vi "myRIO_BRig_FPGA_v3,41__PortC__v2.vi"() -> ()   [LabVIEW 2014]
uses:
  <vilib>/rvi/FXPMathLib/FxpDiv/subVIs/nifxpmath_Div_SimConfig.ctl
  <vilib>/rvi/FXPMathLib/FxpSinAndCos/subVIs/nifxpmath_SinAndCos_SimConfig.ctl
  <vilib>/rvi/FXPMathLib/FxpDiv/simVIs/DllFxpDivTemp_sub.vi
  <vilib>/rvi/FXPMathLib/FxpSinAndCos/simVIs/DllFxpSinAndCosTemp_sub.vi
  <vilib>/rvi/Emulation/niFpgaGetClockAttributes.vi
  <vilib>/rvi/Emulation/niFpgaSctlEmulationGetInTimedLoop.vi
  <vilib>/rvi/Emulation/niFpgaEmulationReportErrorSimple.vi
  <vilib>/rvi/eio/common/nirviEmuTemplateMethod_errors.vi
  <vilib>/rvi/Emulation/niFpgaCriticalErrorInLSC.vi
  <vilib>/rvi/FXPMathLib/FxpDiv/XNode/nifxpmath_Div.xnode
  <vilib>/rvi/FXPMathLib/FxpMul/XNode/nifxpmath_Multiplier.xnode
  <vilib>/rvi/FXPMathLib/FxpSinAndCos/XNode/nifxpmath_SinAndCos.xnode
  <vilib>/rvi/FXPMathLib/FxpSub/XNode/nifxpmath_Sub.xnode
  <vilib>/eio/EIONode/EIONode.xnode
  <vilib>/rvi/FXPMathLib/sim/FxpSim.dll
panel:
  in  "laser_Nshutter":u32=100
  in  "AnaOut_0":i16
  in  "laser_Nvalley":u32=100
  in  "laser_Npeak":u32=100
  in  "laserledMTrig":bool
  in  "laser_selWro_Ntotal":u32=100
  in  "laser_selWro_NDelay":u32
  in  "laser_selRew_Ntotal":u32=100
  in  "laser_selRew_Ndelay":u32
  in  "laserResponse_reward_LED":bool
  in  "laserResponse_wrong_LED":bool
  out "SelectWrong":bool
  out "SelectReward":bool
  in  "laserResponse_wrong":bool
  in  "laserResponse_reward":bool
  in  "Left(F)_or_Right(T)":bool
  in  "ignoreWrong":bool
  in  "SelectionState":bool
  in  "laserMTrig":bool
  in  "FPGA_Stop":bool
  in  "audioTrigger_L":bool
  in  "audioTrigger_R":bool
  in  "audioFreq_L_Hz":u16=1000 min=1000 max=14000 step=1000
  in  "audioAmp_L":u16=1 min=1 max=32767 step=1
  in  "audioFreq_R_Hz":u16=1000 min=1000 max=14000 step=1000
  in  "audioAmp_R":u16=1 min=1 max=32767 step=1
  in  "A3_SL":bool
  in  "A1_SR":bool
  in  "Counts_Reset":bool
  out "A4_LickR":u32
  out "A2_LickL":u32
  in  "A6_Act":bool
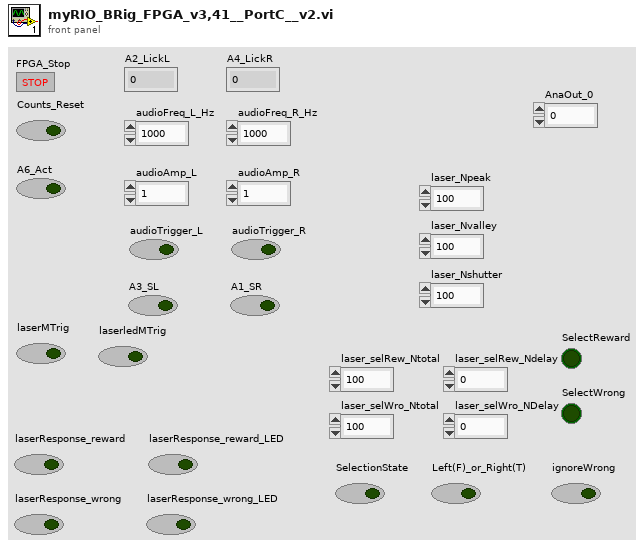
[diagram p1: front panel]
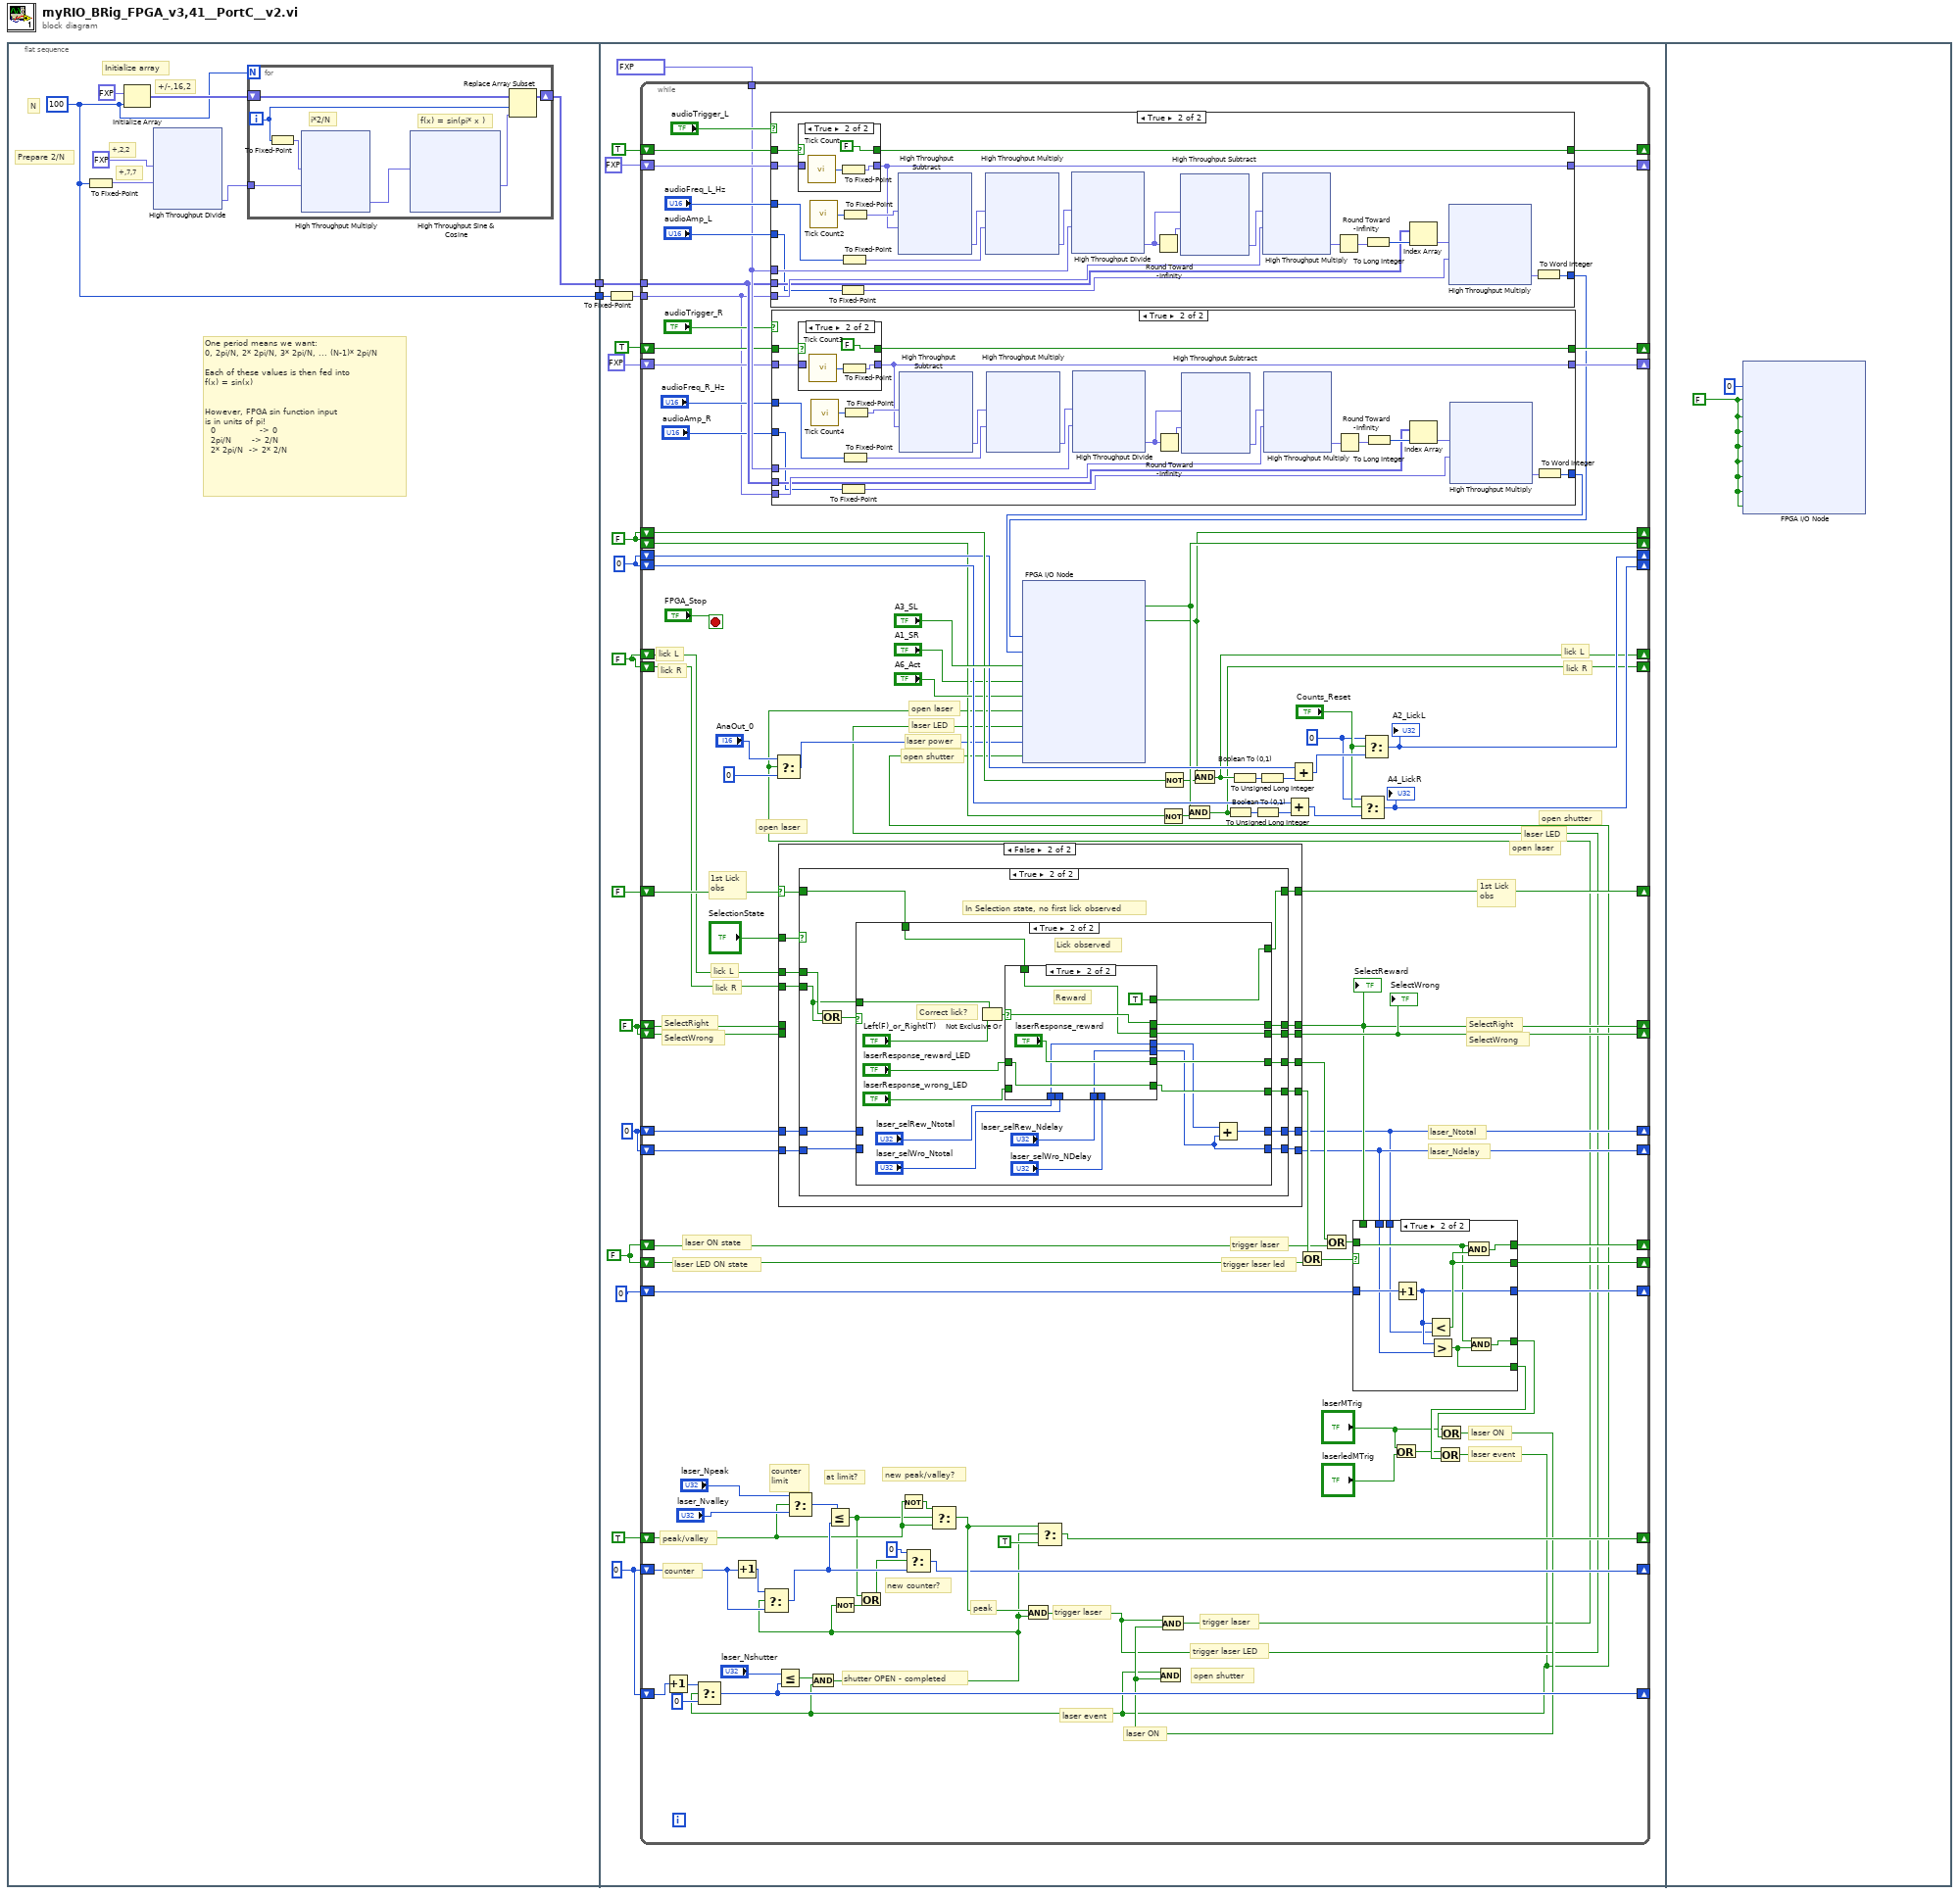
[diagram p0: block diagram]
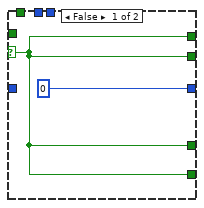
[diagram p2: hidden frame]
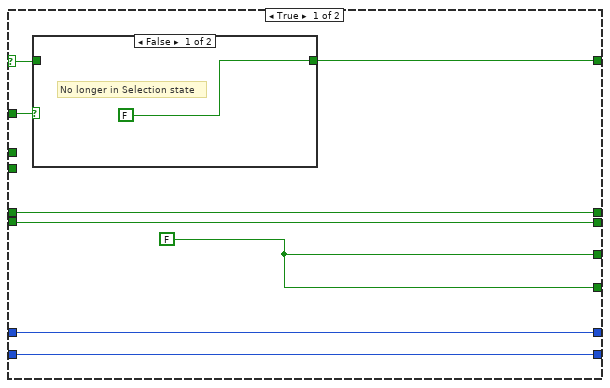
[diagram p3: hidden frame]
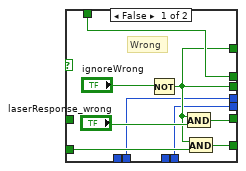
[diagram p7: hidden frame]
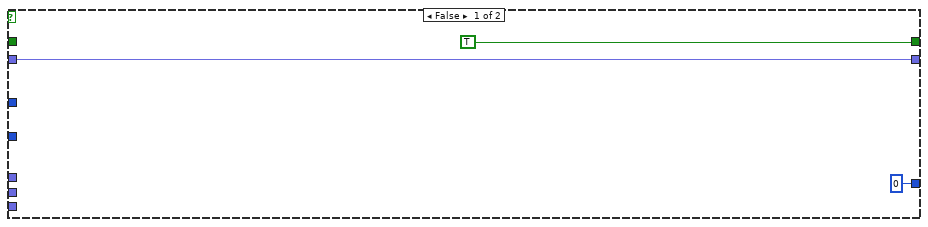
[diagram p8: hidden frame]
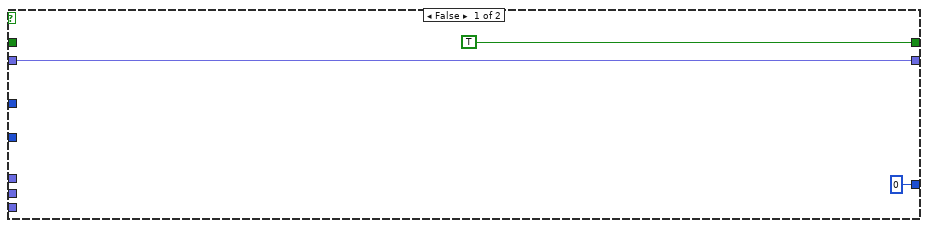
[diagram p10: hidden frame]
diagram:
  n1 = flat-sequence {
    tunnel: [w4] -> w2
    tunnel: [w3] -> w1
    tunnel: w2 -> [w86]
    tunnel: w1 -> [w88]
    frame #0 {
      w3 = 100 ("dimension size")
      # "N"
      # "+,7,7"
      # "+,2,2"
      # "+/-,16,2"
      # "Prepare 2/N"
      # "One period means we want:\n0, 2pi/N, 2* 2pi/N, 3* 2pi/N, ... (N-1)* 2pi/N\n\nEach of these values is then fed into\nf(x) = sin(x)\n\n\nHowever, FPGA sin function input\nis in units of pi!\n  0               -> 0\n  2pi/N       -> 2/N\n  2* 2pi/N  -> 2* 2/N"
      # "Initialize array"
      n2 = To Fixed-Point(number=w3) -> (fixed-point=w6:fxp<+,7,7>)  [unwired: 1 in]
      n3 = Initialize Array(fxp<+/-,16,2> 0.0 ("element"), w3) -> (w9:fxp<+/-,16,2>[])
      n4 = xnode "High Throughput Divide"("x"=fxp<+,2,2> 2.0, "y"=w6) -> ("x/y"=w5:fxp<+,27,0>)
      n5 = for {
        N: w3 -> [_]
        shift-right: [w42] -> w4
        shift-left: w9 -> [w43]
        tunnel: w5 -> [w38]
        i -> [w41]
        # "f(x) = sin(pi* x )"
        # "i*2/N"
        n6 = To Fixed-Point(number=w41) -> (fixed-point=w39:fxp<+,7,7>)  [unwired: 1 in]
        n7 = xnode ("High Throughput Multiply")("x"=w39, "y"=w38) -> ("x*y"=w37:fxp<+,34,7>)
        n8 = xnode "High Throughput Sine & Cosine"("x (pi)"=w37) -> ("sin(x)"=w40:fxp<+/-,16,2>)  [unwired: 1 out]
        n9 = Replace Array Subset(array=w43, new element=w40, index=w41) -> (w42:fxp<+/-,16,2>[])
      }
    }
    frame #1 {
      w74 = u32 0
      w76 = u32 0
      w78 = FALSE
      w77 = FALSE
      w81 = FALSE
      w82 = FALSE
      w83 = u32 0
      n10 = To Fixed-Point(number=w88) -> (fixed-point=w87:fxp<+,7,7>)  [unwired: 1 in]
      n11 = while {
        shift-right: [w186] -> _
        shift-left: TRUE -> [w190]
        shift-right: [w185] -> _
        shift-left: fxp<+,32,32> 0.0 -> [w189]
        tunnel: fxp<+,17,26> 40000000.0 -> [w184]
        tunnel: w87 -> [w177]
        tunnel: w86 -> [w183]
        shift-right: [w176] -> _
        shift-left: TRUE -> [w182]
        shift-right: [w175] -> _
        shift-left: fxp<+,32,32> 0.0 -> [w181]
        shift-right: [w153] -> _
        shift-left: w83 -> [w165]
        shift-right: [w156] -> _
        shift-left: w83 -> [w169]
        shift-right: [w157] -> _
        shift-left: w82 -> [w160]
        shift-right: [w154] -> _
        shift-left: w82 -> [w166]
        shift-right: [w151] -> _
        shift-left: FALSE -> [w150]
        shift-right: [w149] -> _
        shift-left: w81 -> [w147]
        shift-right: [w148] -> _
        shift-left: w81 -> [w146]
        shift-right: [w136] -> _
        shift-left: w77 -> [w138]
        shift-right: [w144] -> _
        shift-left: u32 0 -> [w145]
        shift-right: [w130] -> _
        shift-left: w78 -> [w142]
        shift-right: [w143] -> _
        shift-left: w78 -> [w141]
        shift-right: [w137] -> _
        shift-left: w77 -> [w134]
        shift-right: [w126] -> _
        shift-left: w76 -> [w129]
        shift-right: [w127] -> _
        shift-left: w76 -> [w128]
        shift-right: [w110] -> _
        shift-left: w74 -> [w120]
        shift-right: [w111] -> _
        shift-left: TRUE -> [w114]
        shift-right: [w99] -> _
        shift-left: w74 -> [w103]
        stop <- "FPGA_Stop" stop-if-true
        w162 = u32 0
        # "open shutter"
        # "laser LED"
        # "open laser"
        # "open laser"
        # "trigger laser LED"
        # "trigger laser"
        # "open shutter"
        # "laser ON"
        # "laser power"
        # "open laser"
        # "laser LED"
        # "open shutter"
        # "shutter OPEN - completed"
        # "trigger laser"
        # "peak"
        # "laser event"
        # "new peak/valley?"
        # "counter"
        # "peak/valley"
        # "new counter?"
        # "at limit?"
        # "counter\nlimit"
        # "laser_Ndelay"
        # "laser_Ntotal"
        # "laser event"
        # "laser ON"
        # "laser LED ON state"
        # "laser ON state"
        # "SelectWrong"
        # "SelectRight"
        # "SelectWrong"
        # "SelectRight"
        # "lick R"
        # "lick L"
        # "1st Lick\nobs"
        # "1st Lick\nobs"
        # "lick R"
        # "lick L"
        # "lick R"
        # "lick L"
        # "trigger laser led"
        # "trigger laser"
        n12 = Increment(x=w103) -> (x+1=w102:u32)
        n13 = Increment(x=w120) -> (x+1=w119:u32)
        n14 = case shown="True" "audioTrigger_L" {
          tunnel: w190 -> [_ w365]
          tunnel: w189 -> [w341 w364]
          tunnel: "audioFreq_L_Hz" -> [_ w361]
          tunnel: w184 -> [_ w358]
          tunnel: [w341 w342] -> w185
          tunnel: [TRUE w355] -> w186
          tunnel: w177 -> [_ w354]
          tunnel: w183 -> [_ w349]
          tunnel: "audioAmp_L" -> [_ w347]
          tunnel: [i16 0 w344] -> w172
          frame False {
          }
          frame True {
            n15 = case shown="True" w365 {
              selector: w365 -> [w394 _]
              tunnel: [w394 FALSE] -> w355
              tunnel: w364 -> [w393 _]
              tunnel: [w393 w395] -> w342
              frame False {
              }
              frame True {
                n16 = call "Tick Count"() -> ("Tick Count(Ticks)"=w397:u32)
                n17 = To Fixed-Point(number=w397) -> (fixed-point=w395:fxp<+,32,32>)  [unwired: 1 in]
              }
            }
            n18 = call "Tick Count2"() -> ("Tick Count(Ticks)"=w363:u32)
            n19 = To Fixed-Point(number=w347) -> (fixed-point=w346:fxp<+,15,15>)  [unwired: 1 in]
            n20 = To Fixed-Point(number=w361) -> (fixed-point=w360:fxp<+,14,14>)  [unwired: 1 in]
            n21 = To Fixed-Point(number=w363) -> (fixed-point=w343:fxp<+,32,32>)  [unwired: 1 in]
            n22 = xnode "High Throughput Subtract"("x"=w343, "y"=w342) -> ("x-y"=w362:fxp<+,32,32>)
            n23 = xnode ("High Throughput Multiply")("x"=w362, "y"=w360) -> ("x*y"=w359:fxp<+,46,46>)
            n24 = xnode "High Throughput Divide"("x"=w359, "y"=w358) -> ("x/y"=w357:fxp<+,34,21>)
            n25 = Round Toward -Infinity(1:w357) -> (0:w356:fxp<+,21,21>)
            n26 = xnode "High Throughput Subtract"("x"=w357, "y"=w356) -> ("x-y"=w353:fxp<+,14,1>)
            n27 = xnode ("High Throughput Multiply")("x"=w353, "y"=w354) -> ("x*y"=w350:fxp<+,21,8>)
            n28 = Round Toward -Infinity(1:w350) -> (0:w352:fxp<+,8,8>)
            n29 = To Long Integer(number=w352) -> (32bit integer=w351:i32)
            n30 = Index Array(array=w349, index=w351) -> (element=w348:fxp<+/-,16,2>)
            n31 = xnode ("High Throughput Multiply")("x"=w348, "y"=w346) -> ("x*y"=w345:fxp<+/-,31,17>)
            n32 = To Word Integer(number=w345) -> (16bit integer=w344:i16)
          }
        }
        n33 = case shown="True" "audioTrigger_R" {
          tunnel: w182 -> [_ w306]
          tunnel: w181 -> [w282 w305]
          tunnel: "audioFreq_R_Hz" -> [_ w302]
          tunnel: w184 -> [_ w299]
          tunnel: [w282 w283] -> w175
          tunnel: [TRUE w296] -> w176
          tunnel: w177 -> [_ w295]
          tunnel: w183 -> [_ w290]
          tunnel: "audioAmp_R" -> [_ w288]
          tunnel: [i16 0 w285] -> w173
          frame False {
          }
          frame True {
            n34 = case shown="True" w306 {
              selector: w306 -> [w335 _]
              tunnel: [w335 FALSE] -> w296
              tunnel: w305 -> [w334 _]
              tunnel: [w334 w336] -> w283
              frame False {
              }
              frame True {
                n35 = call "Tick Count3"() -> ("Tick Count(Ticks)"=w338:u32)
                n36 = To Fixed-Point(number=w338) -> (fixed-point=w336:fxp<+,32,32>)  [unwired: 1 in]
              }
            }
            n37 = call "Tick Count4"() -> ("Tick Count(Ticks)"=w304:u32)
            n38 = To Fixed-Point(number=w288) -> (fixed-point=w287:fxp<+,15,15>)  [unwired: 1 in]
            n39 = To Fixed-Point(number=w302) -> (fixed-point=w301:fxp<+,14,14>)  [unwired: 1 in]
            n40 = To Fixed-Point(number=w304) -> (fixed-point=w284:fxp<+,32,32>)  [unwired: 1 in]
            n41 = xnode "High Throughput Subtract"("x"=w284, "y"=w283) -> ("x-y"=w303:fxp<+,32,32>)
            n42 = xnode ("High Throughput Multiply")("x"=w303, "y"=w301) -> ("x*y"=w300:fxp<+,46,46>)
            n43 = xnode "High Throughput Divide"("x"=w300, "y"=w299) -> ("x/y"=w298:fxp<+,34,21>)
            n44 = Round Toward -Infinity(1:w298) -> (0:w297:fxp<+,21,21>)
            n45 = xnode "High Throughput Subtract"("x"=w298, "y"=w297) -> ("x-y"=w294:fxp<+,14,1>)
            n46 = xnode ("High Throughput Multiply")("x"=w294, "y"=w295) -> ("x*y"=w291:fxp<+,21,8>)
            n47 = Round Toward -Infinity(1:w291) -> (0:w293:fxp<+,8,8>)
            n48 = To Long Integer(number=w293) -> (32bit integer=w292:i32)
            n49 = Index Array(array=w290, index=w292) -> (element=w289:fxp<+/-,16,2>)
            n50 = xnode ("High Throughput Multiply")("x"=w289, "y"=w287) -> ("x*y"=w286:fxp<+/-,31,17>)
            n51 = To Word Integer(number=w286) -> (16bit integer=w285:i16)
          }
        }
        n52 = case shown="False" w150 {
          selector: w150 -> [w209 w224]
          tunnel: "SelectionState" -> [w211 w226]
          tunnel: [w210 w225] -> w151
          tunnel: w147 -> [_ w223]
          tunnel: w146 -> [_ w222]
          tunnel: [w208 w221] -> w135
          tunnel: [w206 w220] -> w130
          tunnel: [w207 w219] -> w143
          tunnel: w142 -> [w206 _]
          tunnel: w141 -> [w207 _]
          tunnel: [w208 w218] -> w139
          tunnel: [w205 w217] -> w126
          tunnel: [w204 w216] -> w127
          tunnel: w129 -> [w205 w215]
          tunnel: w128 -> [w204 w214]
          frame True {
            w208 = FALSE
            n53 = case shown="False" w211 {
              tunnel: [FALSE w213] -> w210
              tunnel: w209 -> [_ w213]
              frame False {
                # "No longer in Selection state"
              }
              frame True {
                # "Already observed first lick, no other action"
              }
            }
          }
          frame False {
            n54 = case shown="True" w226 {
              tunnel: [w229 w239] -> w225
              tunnel: w224 -> [w229 w235]
              tunnel: w223 -> [_ w241]
              tunnel: w222 -> [_ w240]
              tunnel: [w229 w238] -> w221
              tunnel: [w229 w237] -> w220
              tunnel: [w229 w236] -> w219
              tunnel: [w229 w234] -> w218
              tunnel: [w228 w233] -> w217
              tunnel: [w227 w232] -> w216
              tunnel: w215 -> [w228 w231]
              tunnel: w214 -> [w227 w230]
              frame False {
                # "Not in Selection state"
              }
              frame True {
                # "In Selection state, no first lick observed"
                n55 = Or(x=w241, y=w240) -> (x .or. y?=w242:bool)
                n56 = case shown="True" w242 {
                  tunnel: w240 -> [_ w262]
                  tunnel: [w245 w255] -> w239
                  tunnel: [w245 w260] -> w238
                  tunnel: [w245 w259] -> w237
                  tunnel: [w245 w258] -> w236
                  tunnel: w235 -> [w245 w257]
                  tunnel: [w245 w256] -> w234
                  tunnel: [w244 w248] -> w233
                  tunnel: [w243 w246] -> w232
                  tunnel: w231 -> [w244 _]
                  tunnel: w230 -> [w243 _]
                  frame False {
                  }
                  frame True {
                    # "Correct lick?"
                    # "Lick observed"
                    n57 = Not Exclusive Or(1:"Left(F)_or_Right(T)", 2:w262) -> (0:w261:bool)
                    n58 = case shown="True" w261 {
                      selector: w261 -> [_ w278]
                      tunnel: [w269 "laserResponse_reward"] -> w260
                      tunnel: [w267 w274] -> w258
                      tunnel: [w271 w278] -> w259
                      tunnel: w257 -> [w271 w274]
                      tunnel: [w268 w276] -> w256
                      tunnel: [w267 TRUE] -> w255
                      tunnel: "laserResponse_reward_LED" -> [_ w276]
                      tunnel: "laserResponse_wrong_LED" -> [w266 _]
                      tunnel: "laser_selRew_Ntotal" -> [_ w273]
                      tunnel: "laser_selWro_Ntotal" -> [w264 _]
                      tunnel: "laser_selRew_Ndelay" -> [_ w275]
                      tunnel: "laser_selWro_NDelay" -> [w265 _]
                      tunnel: [w265 w275] -> w246
                      tunnel: [w264 w273] -> w247
                      frame False {
                        # "Wrong"
                        n59 = Not(x="ignoreWrong") -> (.not. x?=w267:bool)
                        n60 = And(x=w267, y="laserResponse_wrong") -> (x .and. y?=w269:bool)
                        n61 = And(x=w267, y=w266) -> (x .and. y?=w268:bool)
                      }
                      frame True {
                        # "Reward"
                      }
                    }
                    n62 = Add(x=w247, y=w246) -> (x+y=w248:u32)
                  }
                }
              }
            }
          }
        }
        "SelectWrong" <- w143
        "SelectReward" <- w130
        n63 = Select(t="laser_Npeak", s=w114, f="laser_Nvalley") -> (s? t:f=w122:u32)
        n64 = Not(x=w114) -> (.not. x?=w115:bool)
        n65 = Not(x=w160) -> (.not. x?=w159:bool)
        n66 = Not(x=w166) -> (.not. x?=w155:bool)
        n67 = Or(x=w139, y=w138) -> (x .or. y?=w140:bool)
        n68 = Or(x=w135, y=w134) -> (x .or. y?=w133:bool)
        n69 = case shown="True" w140 {
          selector: w140 -> [w193 _]
          tunnel: w145 -> [_ w203]
          tunnel: [u32 0 w200] -> w144
          tunnel: [w193 w201] -> w136
          tunnel: [w193 w202] -> w137
          tunnel: w133 -> [_ w199]
          tunnel: [w193 w198] -> w131
          tunnel: [w193 w197] -> w132
          tunnel: w130 -> [_ _]
          tunnel: w127 -> [_ w196]
          tunnel: w126 -> [_ w195]
          frame False {
          }
          frame True {
            n70 = Increment(x=w203) -> (x+1=w200:u32)
            n71 = Less?(x=w200, y=w195) -> (x < y?=w201:bool)
            n72 = Greater?(x=w200, y=w196) -> (0:w198:bool)
            n73 = And(x=w199, y=w201) -> (x .and. y?=w202:bool)
            n74 = And(x=w199, y=w198) -> (x .and. y?=w197:bool)
          }
        }
        n75 = Or(x="laserMTrig", y="laserledMTrig") -> (x .or. y?=w124:bool)
        n76 = Or(x=w124, y=w131) -> (x .or. y?=w92:bool)
        n77 = Select(t=w102, s=w92, f=u32 0) -> (s? t:f=w99:u32)
        n78 = Less Or Equal?(x="laser_Nshutter", y=w99) -> (x <= y?=w98:bool)
        n79 = And(x=w98, y=w92) -> (x .and. y?=w96:bool)
        n80 = Select(t=w119, s=w96, f=w120) -> (s? t:f=w118:u32)
        n81 = Less Or Equal?(x=w122, y=w118) -> (x <= y?=w108:bool)
        n82 = Not(x=w96) -> (.not. x?=w109:bool)
        n83 = Or(x=w108, y=w109) -> (x .or. y?=w107:bool)
        n84 = Select(t=u32 0, s=w107, f=w118) -> (s? t:f=w110:u32)
        n85 = Select(t=w115, s=w108, f=w114) -> (s? t:f=w113:bool)
        n86 = And(x=w113, y=w96) -> (x .and. y?=w93:bool)
        n87 = Select(t=w113, s=w96, f=TRUE) -> (s? t:f=w111:bool)
        n88 = Or(x="laserMTrig", y=w132) -> (x .or. y?=w95:bool)
        n89 = And(x=w92, y=w95) -> ()  [unwired: 1 out]
        n90 = And(x=w93, y=w95) -> (x .and. y?=w94:bool)
        n91 = Select(t="AnaOut_0", s=w94, f=i16 0) -> (s? t:f=w106:i16)
        n92 = xnode "FPGA I/O Node"("AudioOut/Left"=w172, "AudioOut/Right"=w173, "ConnectorC/DIO3"="A3_SL", "ConnectorC/DIO1"="A1_SR", "ConnectorC/DIO7"="A6_Act", "ConnectorC/DIO0"=w94, "ConnectorC/DIO5"=w93, "ConnectorC/AO0"=w106, "ConnectorC/DIO6"=w92) -> ("ConnectorC/DIO4"=w157:bool, "ConnectorC/DIO2"=w154:bool)  [unwired: 11 in, 11 out]
        n93 = And(x=w157, y=w159) -> (x .and. y?=w148:bool)
        n94 = And(x=w154, y=w155) -> (x .and. y?=w149:bool)
        n95 = Boolean To (0,1)(Boolean=w148) -> (0, 1=w171:i16)
        n96 = Boolean To (0,1)(Boolean=w149) -> (0, 1=w168:i16)
        n97 = To Unsigned Long Integer(number=w171) -> (unsigned 32bit integer=w170:u32)
        n98 = To Unsigned Long Integer(number=w168) -> (unsigned 32bit integer=w167:u32)
        n99 = Add(x=w169, y=w170) -> (x+y=w158:u32)
        n100 = Add(x=w165, y=w167) -> (x+y=w164:u32)
        n101 = Select(t=w162, s="Counts_Reset", f=w158) -> (s? t:f=w156:u32)
        "A4_LickR" <- w156
        n102 = Select(t=w162, s="Counts_Reset", f=w164) -> (s? t:f=w153:u32)
        "A2_LickL" <- w153
      }
    }
    frame #2 {
      w398 = FALSE ("ConnectorA/DIO3")
      n103 = xnode "FPGA I/O Node"("ConnectorC/AO0"=i16 0 ("ConnectorA/AO0"), "ConnectorC/DIO0"=w398, "ConnectorC/DIO1"=w398, "ConnectorC/DIO2"=w398, "ConnectorC/DIO3"=w398, "ConnectorC/DIO4"=w398, "ConnectorC/DIO5"=w398, "ConnectorC/DIO6"=w398, "ConnectorC/DIO7"=w398) -> ()  [unwired: 9 in, 9 out]
    }
  }
